vi "ExSubInitCam.vi"(2 "error in (no error)":errorcluster, 3 "Camera Information":T2={"acquire focus mode"=1, "Exposure"=0.0, "Number of Images"=1, "Software accumulation"=1} {"Software accumulation" min=1; "Number of Images" min=1; "Exposure" format="%.5f"; "acquire focus mode" min=1 max=4 step=1}, 4 "Camera Handle":u32) -> (0 "error out":errorcluster, 1 "Camera Handle":u32)   [LabVIEW 2015]
panel:
  out "Param ID Information":T1 {"Increment" format="%.2f"; "Max Value" format="%.2f"; "Min Value" format="%.2f"; "Default Value" format="%.2f"; "Current Value" format="%.2f"}
  # "ExSubInitCam:\nThis SubVI initializes the camera and \nsets the timing mode and exposure."
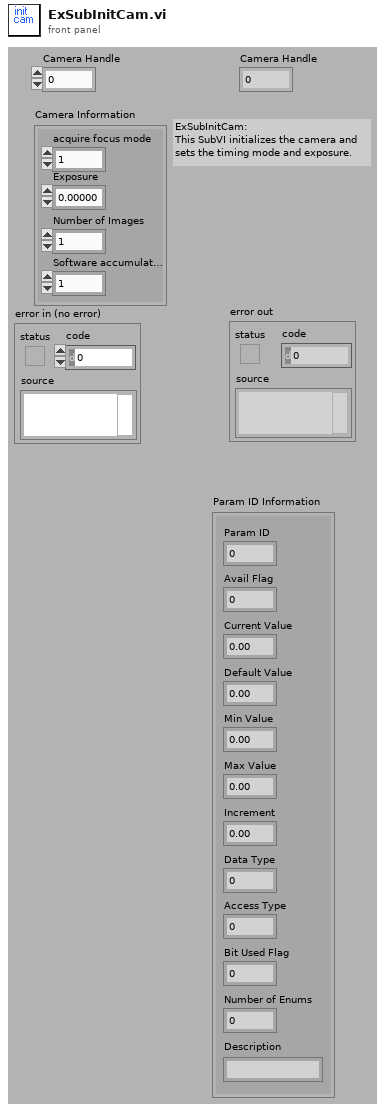
[diagram p1: front panel]
types:
  T1 = cluster{"Param ID":u32, "Avail Flag":u8, "Current Value":dbl, "Default Value":dbl, "Min Value":dbl, "Max Value":dbl, "Increment":dbl, "Data Type":u32, "Access Type":u32, "Bit Used Flag":u32, "Number of Enums":u32, "Description":string}
  T2 = cluster{"acquire focus mode":u32, "Exposure":dbl, "Number of Images":u32, "Software accumulation":u32}
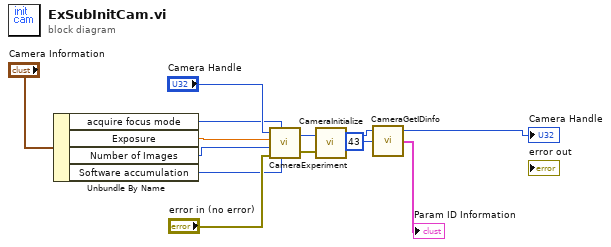
[diagram p0: block diagram]
diagram:
  n1 = Unbundle By Name("Camera Information") -> ("acquire focus mode"=w8:u32, "Exposure"=w7:dbl, "Number of Images"=w6:u32, "Software accumulation"=w5:u32)
  n2 = call <userlib>:"CameraExperiment.vi"("Number of Accumulations"=w5, "Acquire / Focus Flag"=w8, "error in"="error in (no error)", "Number of Images"=w6, "Exposure (sec)"=w7, "Camera Handle"="Camera Handle") -> ("error out"=w9:errorcluster, "Camera Handle"=w10:u32)
  n3 = call <userlib>:"CameraInitialize.vi"("error in"=w9, "Camera Handle"=w10) -> ("Camera Handle"=w4:u32)  [unwired: 1 out]
  n4 = call <userlib>:"CameraGetIDinfo.vi"("Param ID"=u32 43, "Camera handle"=w4) -> ("Param ID Information"=→"Param ID Information":T1, "Camera handle"=→"Camera Handle":u32)  [unwired: 1 in, 1 out]
